vi "All Tests.vi"() -> ()   [LabVIEW 2014]
panel:
  out "XBox":T1
  out "Ultrasonic (in)":dbl
  out "Lift Encoder":T2
  in  "Lift Reset":bool
  out "Arm Beam Breaker":bool
  out "Limit Switches":T3
  in  "Tote in front":bool
  in  "Tote inside":bool
  in  "Camera LED":bool
  out "Distance (ft)":dbl
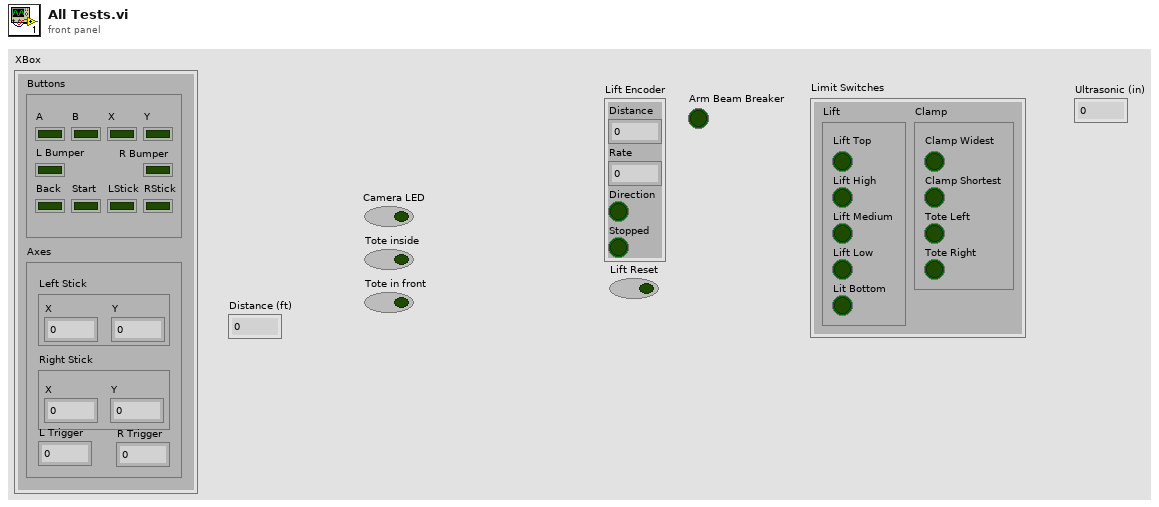
[diagram p1: front panel]
types:
  T1 = cluster{"Buttons":cluster{"A":bool, "B":bool, "X":bool, "Y":bool, "L Bumper":bool, "R Bumper":bool, "Back":bool, "Start":bool, "LStick":bool, "RStick":bool}, "Axes":cluster{"Left Stick":cluster{"X":dbl, "Y":dbl}, "Right Stick":cluster{"X":dbl, "Y":dbl}, "L Trigger":dbl, "R Trigger":dbl}}
  T2 = cluster{"Distance":dbl, "Rate":dbl, "Direction":bool, "Stopped":bool}
  T3 = cluster{"Lift":cluster{"Lift Top":bool, "Lift High":bool, "Lift Medium":bool, "Lift Low":bool, "Lit Bottom":bool}, "Clamp":cluster{"Clamp Widest":bool, "Clamp Shortest":bool, "Tote Left":bool, "Tote Right":bool}}
  T4 = cluster{"Lift":cluster{"Top":bool, "High":bool, "Mid":bool, "Low":bool, "Bot":bool}, "Clamp":cluster{"Widest":bool, "Shortest":bool, "Tote 1":bool, "Tote 2":bool}}
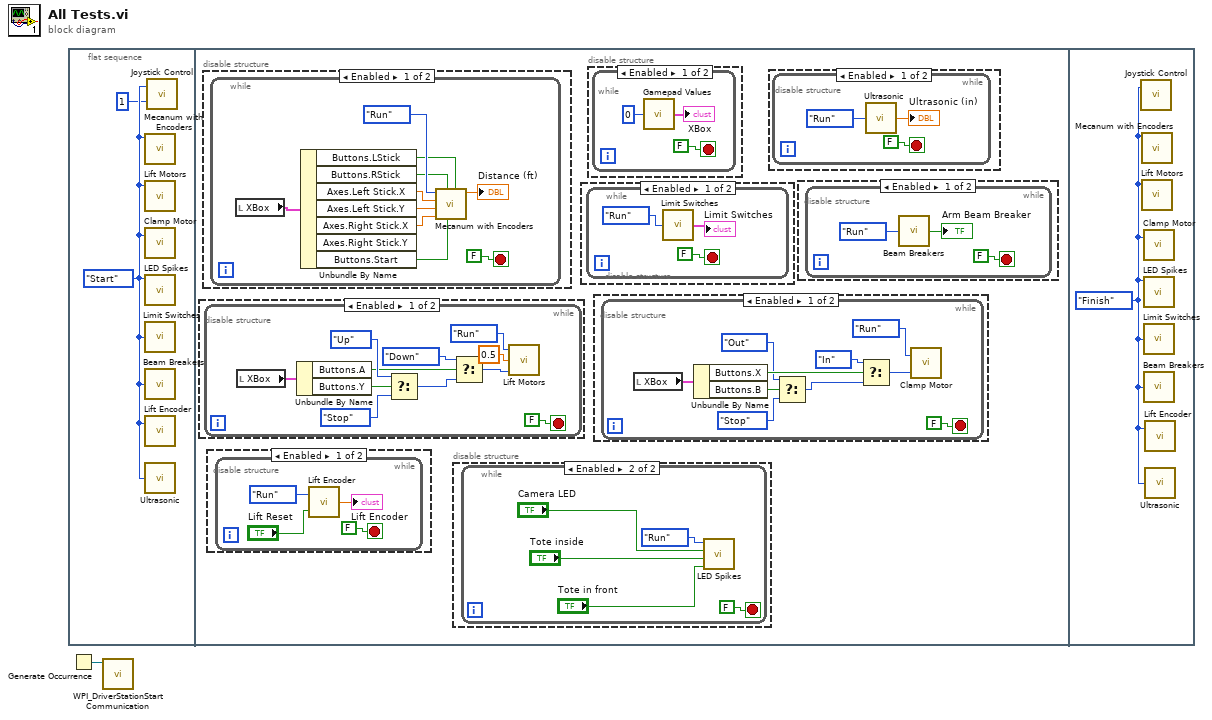
[diagram p0: block diagram]
diagram:
  n1 = flat-sequence {
    frame #0 {
      w3 = enum8{"Start", "Run", "Finish"}."Start" ("Mode")
      n2 = call "Mecanum with Encoders.vi"("Mode"=w3) -> ()  [unwired: 9 in, 1 out]
      n3 = call "Lift Motors.vi"("Mode"=w3) -> ()  [unwired: 2 in]
      n4 = call "Clamp Motor.vi"("Mode"=w3) -> ()  [unwired: 2 in]
      n5 = call "LED Spikes.vi"("Mode"=w3) -> ()  [unwired: 3 in]
      n6 = call "Limit Switches.vi"("Mode"=w3) -> ()  [unwired: 1 out]
      n7 = call "Beam Breakers.vi"("Mode"=w3) -> ()  [unwired: 1 out]
      n8 = call "Lift Encoder.vi"("Mode"=w3) -> ()  [unwired: 1 in, 1 out]
      n9 = call "Ultrasonic.vi"("Mode"=w3) -> ()  [unwired: 1 out]
      n10 = call "Joystick Control.vi"("Number of Joysticks"=1, "Mode"=w3) -> ()  [unwired: 1 out]
    }
    frame #1 {
      n11 = disable-structure shown="Enabled" {
        frame Enabled {
          n12 = while {
            stop <- FALSE stop-if-true
            n13 = local read "XBox"() -> (w12:T1)
            n14 = Unbundle By Name(w12) -> ("Buttons.A"=w6:bool, "Buttons.Y"=w5:bool)
            n15 = Select(t=enum16{"Stop", "Up", "Down"}."Up" ("Direction"), s=w5, f=enum16{"Stop", "Up", "Down"}."Stop" ("Direction")) -> (s? t:f=w9:enum16{"Stop", "Up", "Down"})
            n16 = Select(t=enum16{"Stop", "Up", "Down"}."Down" ("Direction"), s=w6, f=w9) -> (s? t:f=w7:enum16{"Stop", "Up", "Down"})
            n17 = call "Lift Motors.vi"("Direction"=w7, "Speed"=0.5, "Mode"=enum8{"Start", "Run", "Finish"}."Run") -> ()
          }
        }
        frame Disabled {
        }
      }
      n18 = disable-structure shown="Enabled" {
        frame Enabled {
          n19 = while {
            stop <- FALSE stop-if-true
            n20 = local read "XBox"() -> (w52:T1)
            n21 = Unbundle By Name(w52) -> ("Buttons.LStick"=w46:bool, "Buttons.RStick"=w48:bool, "Axes.Left Stick.X"=w51:dbl, "Axes.Left Stick.Y"=w50:dbl, "Axes.Right Stick.X"=w49:dbl, "Buttons.Start"=w47:bool)  [unwired: 1 out]
            n22 = call "Mecanum with Encoders.vi"("Slow?"=w46, "Reset"=w47, "Fast?"=w48, "Turn"=w49, "Forward/Backward"=w50, "Strafe"=w51, "Mode"=enum8{"Start", "Run", "Finish"}."Run") -> ("Distance (ft)"=→"Distance (ft)":dbl)  [unwired: 3 in]
          }
        }
        frame Disabled {
        }
      }
      n23 = disable-structure shown="Enabled" {
        frame Enabled {
          n24 = while {
            stop <- FALSE stop-if-true
            n25 = call "Lift Encoder.vi"("Reset"="Lift Reset", "Mode"=enum8{"Start", "Run", "Finish"}."Run") -> ("Lift Distance"=→"Lift Encoder":dbl)
          }
        }
        frame Disabled {
        }
      }
      n26 = disable-structure shown="Enabled" {
        frame Disabled {
        }
        frame Enabled {
          n27 = while {
            stop <- FALSE stop-if-true
            n28 = call "LED Spikes.vi"("Tote in front LED"="Tote in front", "Tote inside LED"="Tote inside", "Camera LED"="Camera LED", "Mode"=enum8{"Start", "Run", "Finish"}."Run") -> ()
          }
        }
      }
      n29 = disable-structure shown="Enabled" {
        frame Enabled {
          n30 = while {
            stop <- FALSE stop-if-true
            n31 = call "Limit Switches.vi"("Mode"=enum8{"Start", "Run", "Finish"}."Run") -> ("Limit Switches"=→"Limit Switches":T4)
          }
        }
        frame Disabled {
        }
      }
      n32 = disable-structure shown="Enabled" {
        frame Enabled {
          n33 = while {
            stop <- FALSE stop-if-true
            n34 = call "Gamepad Values.vi"("Index"=0) -> ("XBox"=→"XBox":T1)
          }
        }
        frame Disabled {
        }
      }
      n35 = disable-structure shown="Enabled" {
        frame Enabled {
          n36 = while {
            stop <- FALSE stop-if-true
            n37 = local read "XBox"() -> (w22:T1)
            n38 = Unbundle By Name(w22) -> ("Buttons.X"=w21:bool, "Buttons.B"=w20:bool)
            n39 = Select(t=enum16{"Stop", "In", "Out"}."Out" ("Direction"), s=w20, f=enum16{"Stop", "In", "Out"}."Stop" ("Direction")) -> (s? t:f=w18:enum16{"Stop", "In", "Out"})
            n40 = Select(t=enum16{"Stop", "In", "Out"}."In" ("Direction"), s=w21, f=w18) -> (s? t:f=w15:enum16{"Stop", "In", "Out"})
            n41 = call "Clamp Motor.vi"("Direction"=w15, "Mode"=enum8{"Start", "Run", "Finish"}."Run") -> ()  [unwired: 1 in]
          }
        }
        frame Disabled {
        }
      }
      n42 = disable-structure shown="Enabled" {
        frame Enabled {
          n43 = while {
            stop <- FALSE stop-if-true
            n44 = call "Ultrasonic.vi"("Mode"=enum16{"Start", "Run", "Finish"}."Run" ("State")) -> ("Distance (in)"=→"Ultrasonic (in)":dbl)
          }
        }
        frame Disabled {
        }
      }
      n45 = disable-structure shown="Enabled" {
        frame Enabled {
          n46 = while {
            stop <- FALSE stop-if-true
            n47 = call "Beam Breakers.vi"("Mode"=enum8{"Start", "Run", "Finish"}."Run") -> ("Clamp Beam Breaker"=→"Arm Beam Breaker":bool)
          }
        }
        frame Disabled {
        }
      }
    }
    frame #2 {
      w56 = enum8{"Start", "Run", "Finish"}."Finish" ("Mode")
      n48 = call "Joystick Control.vi"("Mode"=w56) -> ()  [unwired: 1 in, 1 out]
      n49 = call "Mecanum with Encoders.vi"("Mode"=w56) -> ()  [unwired: 9 in, 1 out]
      n50 = call "Lift Motors.vi"("Mode"=w56) -> ()  [unwired: 2 in]
      n51 = call "Clamp Motor.vi"("Mode"=w56) -> ()  [unwired: 2 in]
      n52 = call "LED Spikes.vi"("Mode"=w56) -> ()  [unwired: 3 in]
      n53 = call "Limit Switches.vi"("Mode"=w56) -> ()  [unwired: 1 out]
      n54 = call "Beam Breakers.vi"("Mode"=w56) -> ()  [unwired: 1 out]
      n55 = call "Lift Encoder.vi"("Mode"=w56) -> ()  [unwired: 1 in, 1 out]
      n56 = call "Ultrasonic.vi"("Mode"=w56) -> ()  [unwired: 1 out]
    }
  }
  n57 = Generate Occurrence() -> (w1:refnum<k4>)
  n58 = call <vilib>:"WPI_DriverStationStart Communication.vi"("occurrence"=w1) -> ()  [unwired: 11 in]
